vi "Fetch (NT).vi"(7 "PV name":string, 8 "error in":errorcluster, 10 "default value":refnum<class "NT Base.lvclass">, 11 "Server in":refnum<class "Server.lvclass">) -> (0 "error out":errorcluster, 2 "value":refnum<class "NT Base.lvclass">, 3 "Server out":refnum<class "Server.lvclass">)   [LabVIEW 2020, in "PV Access.lvlib" / "PVA Server.lvlib" / "Server.lvclass"]
uses:
  Server.lvclass
  Server.lvclass/Server.ctl
  Source/Source.lvclass
  PV Data/PV Data/PV Data.lvclass
  PV Data/NT Base/NT Base.lvclass
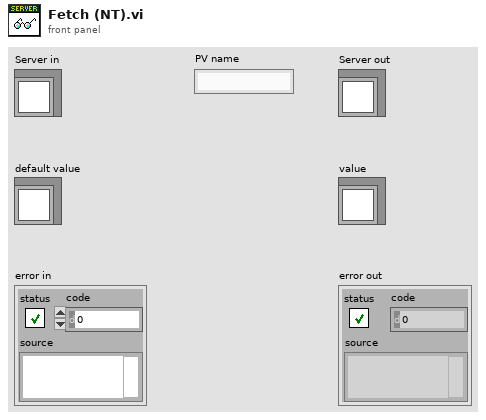
[diagram p1: front panel]
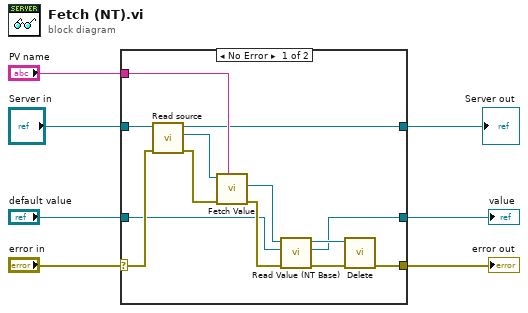
[diagram p0: block diagram]
diagram:
  n1 = case shown="No Error" "error in" {
    selector: "error in" -> [w19 w22]
    tunnel: [w11 w22] -> w7
    tunnel: "PV name" -> [w20 _]
    tunnel: "Server in" -> [w17 w23]
    tunnel: [w16 w23] -> w3
    tunnel: "default value" -> [w9 w21]
    tunnel: [w8 w21] -> w1
    frame No Error {
      n2 = call "Read source.vi"("error in (no error)"=w19, "Server in"=w17) -> ("error out"=w18:errorcluster, "Source"=w15:refnum<class "Source.lvclass">, "Server out"=w16:refnum<class "Server.lvclass">)  [unwired: 7 in]
      n3 = call "Fetch Value.vi"("PV name"=w20, "error in"=w18, "Source in"=w15) -> ("error out"=w10:errorcluster, "PV Data out"=w14:refnum<class "PV Data.lvclass">)  [unwired: 6 in, 1 out]
      n4 = call "Read Value (NT Base).vi"("error in (no error)"=w10, "default value"=w9, "PV Data in"=w14) -> ("error out"=w13:errorcluster, "value"=w8:refnum<class "NT Base.lvclass">, "PV Data out"=w12:refnum<class "PV Data.lvclass">)  [unwired: 6 in]
      n5 = call "Delete.vi"("error in (no error)"=w13, "PV Data in"=w12) -> ("error out"=w11:errorcluster)  [unwired: 9 in]
    }
    frame Error {
    }
  }
  "Server out" <- w3
  "error out" <- w7
  "value" <- w1
